vi "generateTelemetryFPGAData.vi"(8 "error in (no error)":errorcluster, 10 "TelemetryFPGAData":T1, 11 "UserEvents in":refnum<class "UserEvents.lvclass">) -> (0 "error out":errorcluster, 3 "UserEvents out":refnum<class "UserEvents.lvclass">)   [LabVIEW 2016, in "UserEvents.lvclass"]
uses:
  UserEvents.lvclass
  DataTypes/Topics/TelemetryFPGAData.ctl
  DataTypes/Topics/Parts/Timestamp.ctl
  UserEvents.lvclass/UserEvents.ctl
  DataTypes/Topics/M1M3SupportTopics.lvlib
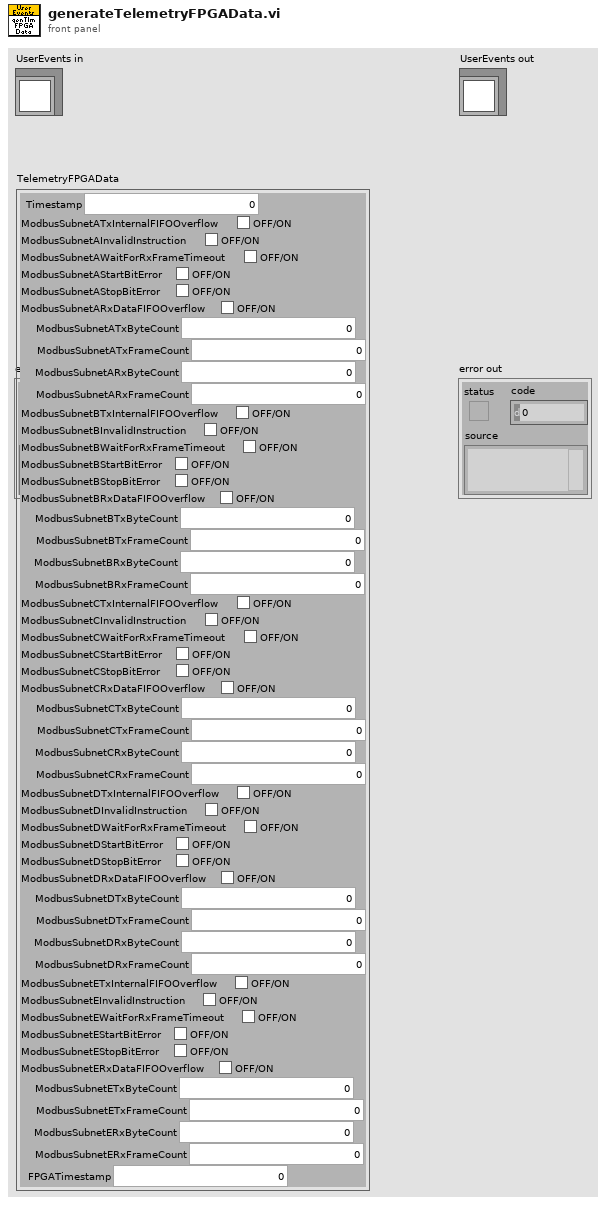
[diagram p1: front panel]
types:
  T1 = typedef "M1M3SupportTopics.lvlib/TelemetryFPGAData.ctl" = cluster{"Timestamp":T2, "ModbusSubnetATxInternalFIFOOverflow":bool, "ModbusSubnetAInvalidInstruction":bool, "ModbusSubnetAWaitForRxFrameTimeout":bool, "ModbusSubnetAStartBitError":bool, "ModbusSubnetAStopBitError":bool, "ModbusSubnetARxDataFIFOOverflow":bool, "ModbusSubnetATxByteCount":u32, "ModbusSubnetATxFrameCount":u32, "ModbusSubnetARxByteCount":u32, "ModbusSubnetARxFrameCount":u32, "ModbusSubnetBTxInternalFIFOOverflow":bool, "ModbusSubnetBInvalidInstruction":bool, "ModbusSubnetBWaitForRxFrameTimeout":bool, "ModbusSubnetBStartBitError":bool, "ModbusSubnetBStopBitError":bool, "ModbusSubnetBRxDataFIFOOverflow":bool, "ModbusSubnetBTxByteCount":u32, "ModbusSubnetBTxFrameCount":u32, "ModbusSubnetBRxByteCount":u32, "ModbusSubnetBRxFrameCount":u32, "ModbusSubnetCTxInternalFIFOOverflow":bool, "ModbusSubnetCInvalidInstruction":bool, "ModbusSubnetCWaitForRxFrameTimeout":bool, "ModbusSubnetCStartBitError":bool, "ModbusSubnetCStopBitError":bool, "ModbusSubnetCRxDataFIFOOverflow":bool, "ModbusSubnetCTxByteCount":u32, "ModbusSubnetCTxFrameCount":u32, "ModbusSubnetCRxByteCount":u32, "ModbusSubnetCRxFrameCount":u32, "ModbusSubnetDTxInternalFIFOOverflow":bool, "ModbusSubnetDInvalidInstruction":bool, "ModbusSubnetDWaitForRxFrameTimeout":bool, "ModbusSubnetDStartBitError":bool, "ModbusSubnetDStopBitError":bool, "ModbusSubnetDRxDataFIFOOverflow":bool, "ModbusSubnetDTxByteCount":u32, "ModbusSubnetDTxFrameCount":u32, "ModbusSubnetDRxByteCount":u32, "ModbusSubnetDRxFrameCount":u32, "ModbusSubnetETxInternalFIFOOverflow":bool, "ModbusSubnetEInvalidInstruction":bool, "ModbusSubnetEWaitForRxFrameTimeout":bool, "ModbusSubnetEStartBitError":bool, "ModbusSubnetEStopBitError":bool, "ModbusSubnetERxDataFIFOOverflow":bool, "ModbusSubnetETxByteCount":u32, "ModbusSubnetETxFrameCount":u32, "ModbusSubnetERxByteCount":u32, "ModbusSubnetERxFrameCount":u32, "FPGATimestamp":dbl}
  T2 = typedef "M1M3SupportTopics.lvlib/Timestamp.ctl" = dbl
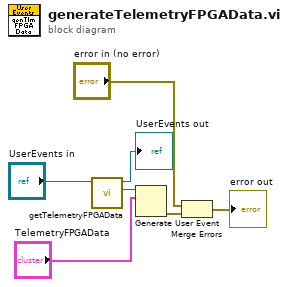
[diagram p0: block diagram]
diagram:
  n1 = call "getTelemetryFPGAData.vi"("UserEvents in"="UserEvents in") -> ("TelemetryFPGAData"=w7:refnum<user-event>, "UserEvents out"=→"UserEvents out":refnum<class "UserEvents.lvclass">)  [unwired: 9 in]
  n2 = Generate User Event(user event=w7, event data cluster="TelemetryFPGAData") -> (error out=w3:errorcluster)  [unwired: 2 in, 1 out]
  n3 = Merge Errors("error in (no error)", w3) -> (→"error out":errorcluster)
